vi "Megnyitás.vi"(8 "error in":errorcluster) -> (0 "error out":errorcluster, 3 "Felhasználói adatok out":string[][](array[string]))   [LabVIEW 2014]
panel:
  out "text":string
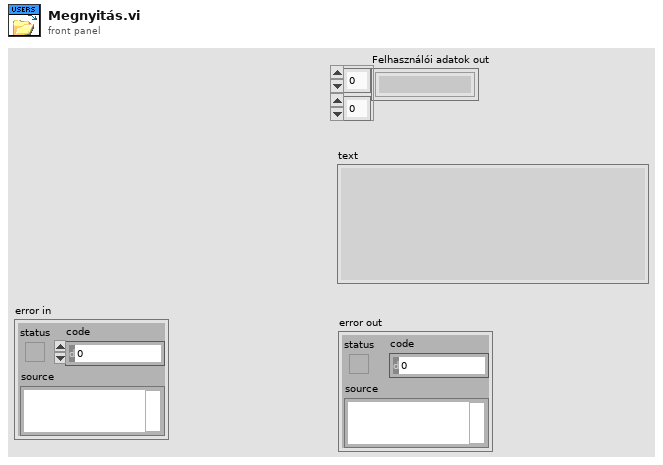
[diagram p1: front panel]
types:
  T1 = typedef "Felhasználó típus.ctl" = cluster{"NÉV:":string, "Jelszó: (csak számjegyek)":string, "Felhasználói szint":string}
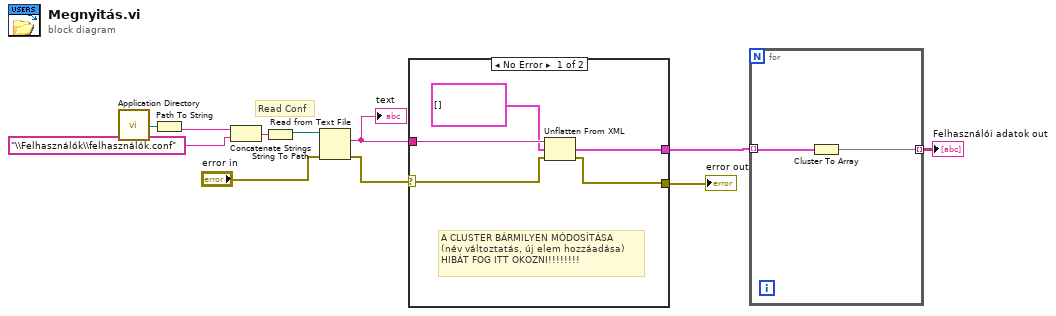
[diagram p0: block diagram]
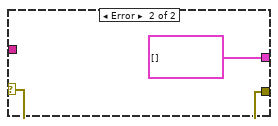
[diagram p2: hidden frame]
diagram:
  # "Read Conf"
  n1 = call <vilib>:"Application Directory.vi"() -> ("Application Directory"=w7:path)
  n2 = Path To String(path=w7) -> (string=w5:string)
  n3 = Concatenate Strings(w5, "\\Felhasználók\\felhasználók.conf" ("prompt (Choose or enter file path)")) -> (w6:string)
  n4 = String To Path(string=w6) -> (path=w3:path)
  n5 = Read from Text File(file (use dialog)=w3, error in="error in") -> (text=w11:string, error out=w10:errorcluster)  [unwired: 2 in, 2 out]
  "text" <- w11
  n6 = case shown="No Error" w10 {
    selector: w10 -> [w14 w18]
    tunnel: w11 -> [w16 _]
    tunnel: [w15 T1[] []] -> w2
    tunnel: [w13 w18] -> w9
    frame No Error {
      # "A CLUSTER BÁRMILYEN MÓDOSÍTÁSA\n(név változtatás, új elem hozzáadása)\nHIBÁT FOG ITT OKOZNI!!!!!!!!"
      n7 = Unflatten From XML(xml string=w16, type=T1[] [], error in (no error)=w14) -> (value=w15:T1[], error out=w13:errorcluster)
    }
    frame Error {
    }
  }
  "error out" <- w9
  n8 = for {
    tunnel: w2 -> [w20] mode=indexing
    tunnel: [w19] -> w1 mode=indexing
    n9 = Cluster To Array(cluster=w20) -> (array=w19:string[])
  }
  "Felhasználói adatok out" <- w1
